vi "EJEM12.vi"   [LabVIEW 2013]
types:
  T1 = enum16{"open", "replace", "create", "open or create", "replace or create", "replace or create with confirmation"}
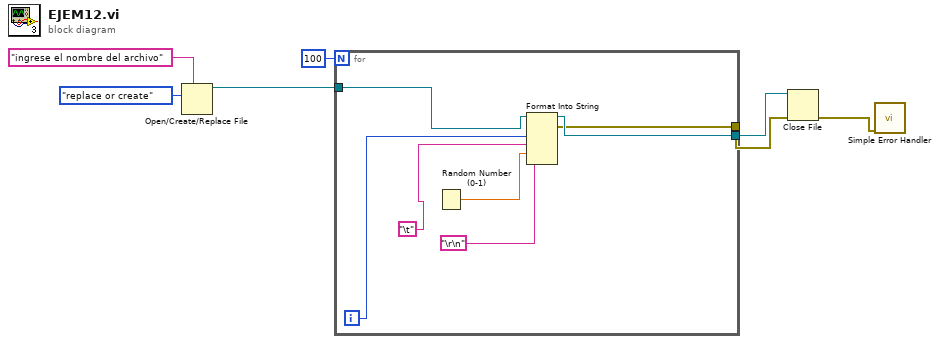
[diagram p0: block diagram]
diagram:
  n1 = Open/Create/Replace File(prompt="ingrese el nombre del archivo", operation (0:open)=T1."replace or create") -> (refnum out=w4:refnum<file>)  [unwired: 4 in, 2 out]
  n2 = for {
    N: 100 -> [_]
    tunnel: w4 -> [w14]
    tunnel: [w9] -> w3
    tunnel: [w8] -> w2
    i -> [w13]
    n3 = Random Number (0-1)() -> (number: 0 to 1=w11:dbl)
    n4 = Format Into String(initial string=w14, w13, "\t", w11, "\r\n") -> (resulting string=w9:refnum<file>, error out=w8:errorcluster)  [unwired: 2 in]
  }
  n5 = Close File(refnum=w3, error in=w2) -> (error out=w1:errorcluster)  [unwired: 1 out]
  n6 = call <vilib>:"Simple Error Handler.vi"("error in (no error)"=w1) -> ()  [unwired: 4 in, 5 out]
